vi "加法.vi"(1 "b":dbl, 2 "a":dbl) -> (0 "c":dbl)   [LabVIEW 2014]
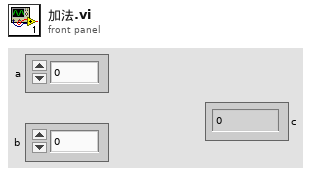
[diagram p1: front panel]
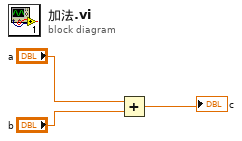
[diagram p0: block diagram]
diagram:
  n1 = Add(x="a", y="b") -> (x+y=→"c":dbl)
